vi "FGV_stringBuffer.vi"(7 "Enum":T1, 8 "error in":errorcluster, 10 "String In":string) -> (0 "error out":errorcluster, 2 "String Out":string)   [LabVIEW 2023]
uses:
  enumFGVstringBuffer.ctl
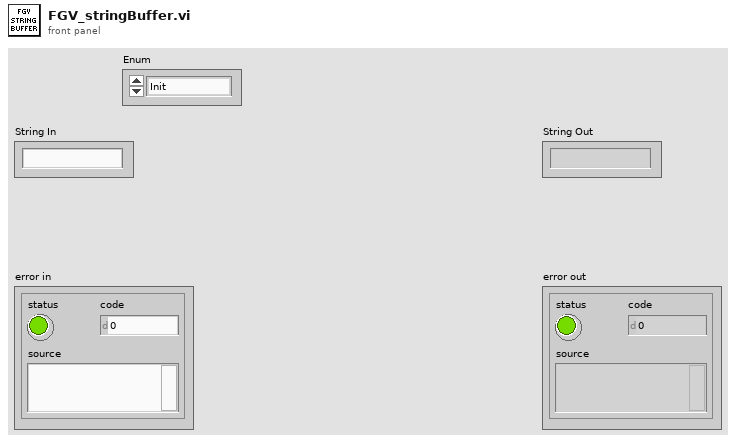
[diagram p1: front panel]
types:
  T1 = typedef "enumFGVstringBuffer.ctl" = enum16{"Init", "Write", "Read"}
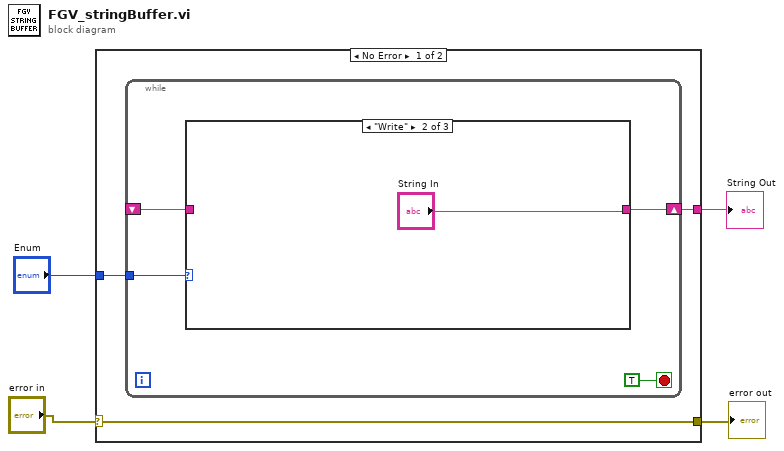
[diagram p0: block diagram]
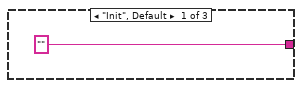
[diagram p2: hidden frame]
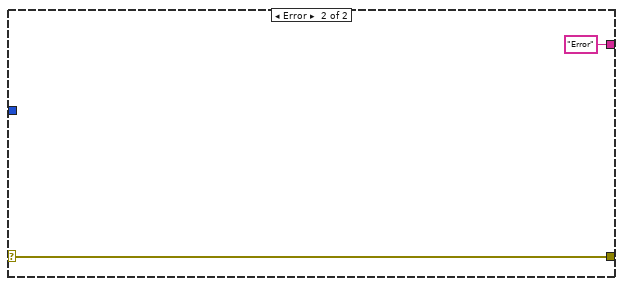
[diagram p4: hidden frame]
diagram:
  n1 = case shown="No Error" "error in" {
    selector: "error in" -> [w5 w16]
    tunnel: "Enum" -> [w7 _]
    tunnel: [w6 "Error" ("String In")] -> w3
    tunnel: [w5 w16] -> w1
    frame No Error {
      n2 = while {
        tunnel: w7 -> [w10]
        shift-right: [w9] -> w6
        shift-left: _ -> [w8]
        stop <- TRUE stop-if-true
        n3 = case shown="\"Write\"" w10 {
          tunnel: ["" ("String In") "String In" w14] -> w9
          tunnel: w8 -> [_ _ w14]
          frame "Init", Default {
          }
          frame "Write" {
          }
          frame "Read" {
          }
        }
      }
    }
    frame Error {
    }
  }
  "String Out" <- w3
  "error out" <- w1
